vi "PDE Thermal Distribution_Gen RHS Plot.vi"(9 "Y":T1={"start y"=0.0, "end y"=1.0, "# of y-points"=11}, 10 "X":T2={"start x"=0.0, "end x"=1.0, "# of x-points"=11}, 11 "RHS Para":T3) -> (3 "RHS":dbl[][](graph))   [LabVIEW 2023]
doc: "Generate RHS plot for PDE Thermal Distribution.vi example."
uses:
  <vilib>/Analysis/1siggen.llb/Ramp Pattern by Samples.vi
  <vilib>/Analysis/NI_AALBase.lvlib
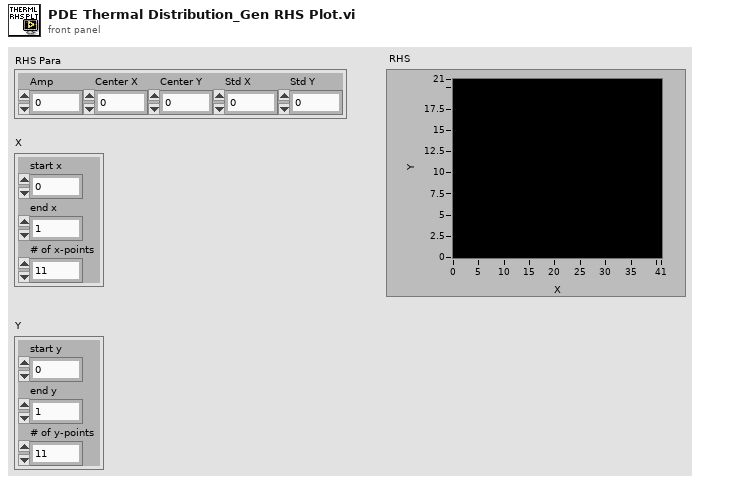
[diagram p1: front panel]
types:
  T1 = cluster{"start y":dbl, "end y":dbl, "# of y-points":i32}
  T2 = cluster{"start x":dbl, "end x":dbl, "# of x-points":i32}
  T3 = cluster{"Amp":dbl, "Center X":dbl, "Center Y":dbl, "Std X":dbl, "Std Y":dbl}
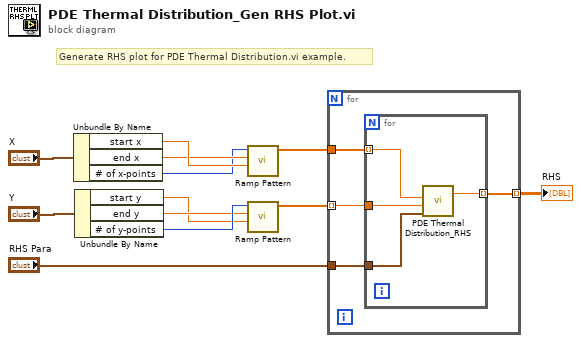
[diagram p0: block diagram]
diagram:
  # "Generate RHS plot for PDE Thermal Distribution.vi example."
  n1 = Unbundle By Name("X") -> ("start x"=w9:dbl, "end x"=w8:dbl, "# of x-points"=w7:i32)
  n2 = Unbundle By Name("Y") -> ("start y"=w10:dbl, "end y"=w11:dbl, "# of y-points"=w12:i32)
  n3 = call-poly <vilib>:"Ramp Pattern.vi"("start"=w9, "end"=w8, "samples"=w7) -> ("Ramp Pattern"=w5:dbl[])  [unwired: 7 in, 1 out]
  n4 = call-poly <vilib>:"Ramp Pattern.vi"("start"=w10, "end"=w11, "samples"=w12) -> ("Ramp Pattern"=w6:dbl[])  [unwired: 7 in, 1 out]
  n5 = for {
    tunnel: w6 -> [w15] mode=indexing
    tunnel: w5 -> [w16]
    tunnel: [w14] -> w4 mode=indexing
    tunnel: "RHS Para" -> [w13]
    n6 = for {
      tunnel: w16 -> [w17] mode=indexing
      tunnel: w15 -> [w18]
      tunnel: [w20] -> w14 mode=indexing
      tunnel: w13 -> [w19]
      n7 = call "PDE Thermal Distribution_RHS.vi"("data"=w19, "y"=w18, "x"=w17) -> ("F(t, x, y)"=w20:dbl)  [unwired: 1 in, 1 out]
    }
  }
  "RHS" <- w4
